vi "Calc_3-Ball-Conveyor_Module.vi"(0 "Enable":bool, 5 "Reset":bool, 7 "Grab Sensor":bool, 9 "Bottom Sensor":bool, 11 "Ball in Turret":bool=TRUE, 12 "Ball is out":bool) -> (4 "Motor Speed":dbl, 6 "Accepting Balls":bool, 8 "State":T1=enum."Holding 2", 10 "Ball Count":i32=2)   [LabVIEW 2012]
uses:
  3-Ball-Conveyor_Module_State.ctl
panel:
  in  "Slow":dbl=0.3
  in  "Fast":dbl=0.6
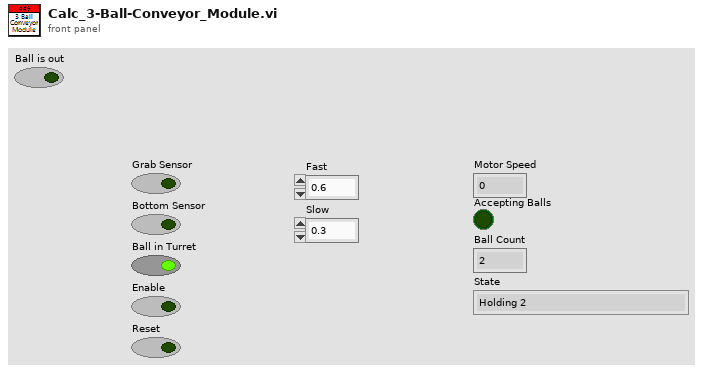
[diagram p1: front panel]
types:
  T1 = typedef "3-Ball-Conveyor_Module_State.ctl" = enum16{"No Balls", "Collecting Ball", "Holding 1", "Pushing Ball Out", "Holding 2", "Lowering Ball", "Reset", "Disabled"}
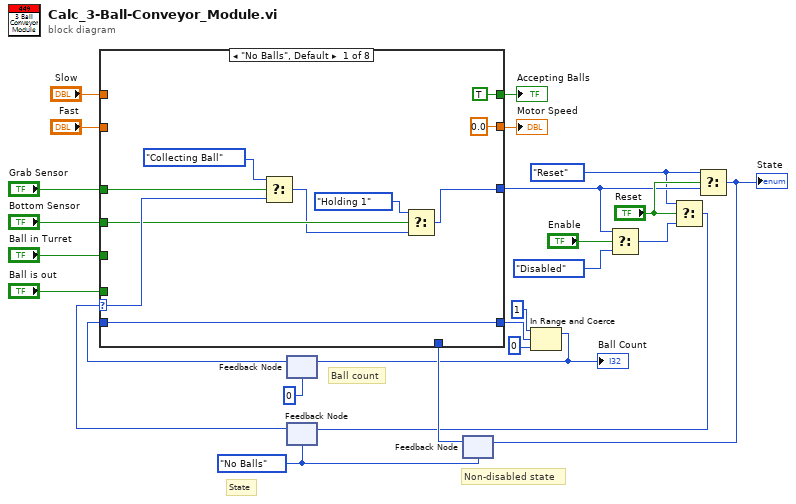
[diagram p0: block diagram]
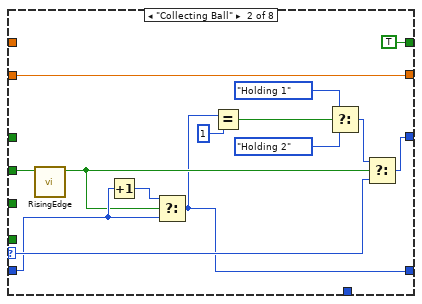
[diagram p2: hidden frame]
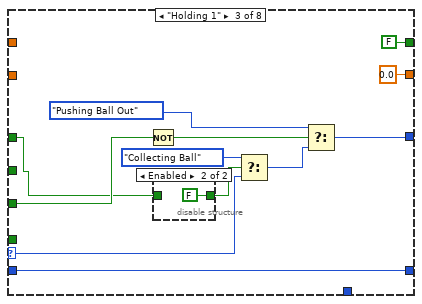
[diagram p3: hidden frame]
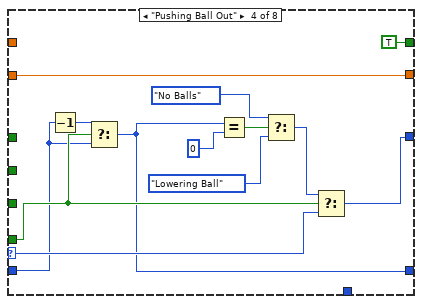
[diagram p5: hidden frame]
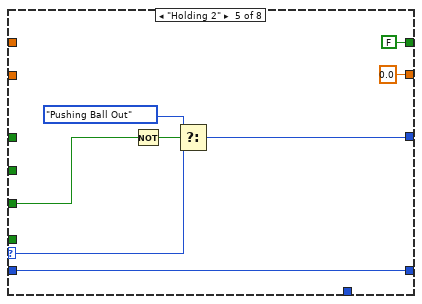
[diagram p6: hidden frame]
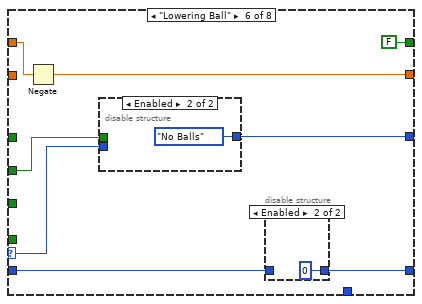
[diagram p7: hidden frame]
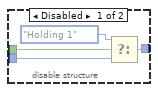
[diagram p8: hidden frame]
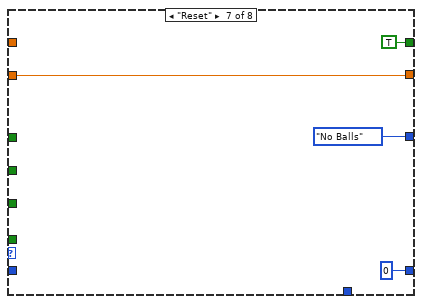
[diagram p10: hidden frame]
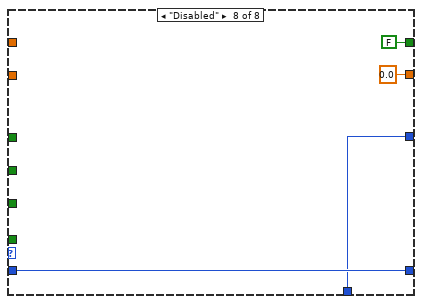
[diagram p11: hidden frame]
diagram:
  w6 = 3-Ball-Conveyor_Module_State."Reset"
  w11 = 3-Ball-Conveyor_Module_State."No Balls"
  # "Ball count"
  # "Non-disabled state"
  # "State"
  n1 = feedback #1(0) -> (w17:i32)
  n2 = feedback #2(w11) -> (w25:T1)
  n3 = feedback #3(w11) -> (w10:T1)
  n4 = case shown="\"No Balls\", Default" w25 {
    selector: w25 -> [w34 w46 w53 w74 w80 w88 _ _]
    tunnel: [0.0 ("Fast") w49 0.0 ("Fast") w76 0.0 ("Fast") w91 w103 0.0 ("Fast")] -> w24
    tunnel: [TRUE TRUE FALSE TRUE FALSE FALSE TRUE FALSE] -> w23
    tunnel: "Grab Sensor" -> [w35 _ w51 _ _ _ _ _]
    tunnel: [w26 w42 w59 w70 w81 w89 3-Ball-Conveyor_Module_State."No Balls" w104] -> w9
    tunnel: "Fast" -> [_ w49 _ w76 _ _ w103 _]
    tunnel: "Bottom Sensor" -> [w29 w47 _ _ _ w85 _ _]
    tunnel: "Ball in Turret" -> [_ _ w57 _ w82 _ _ _]
    tunnel: w17 -> [w31 w41 w56 w65 w79 w86 _ w105]
    tunnel: [w31 w36 w56 w64 w79 w87 0 ("t") w105] -> w4
    tunnel: "Slow" -> [_ _ _ _ _ w92 _ _]
    tunnel: w10 -> [_ _ _ _ _ _ _ w104]
    tunnel: "Ball is out" -> [_ _ _ w66 _ _ _ _]
    frame "No Balls", Default {
      n5 = Select(t=3-Ball-Conveyor_Module_State."Collecting Ball", s=w35, f=w34) -> (s? t:f=w28:T1)
      n6 = Select(t=3-Ball-Conveyor_Module_State."Holding 1", s=w29, f=w28) -> (s? t:f=w26:T1)
    }
    frame "Collecting Ball" {
      n7 = call "RisingEdge.vi"("BooleanIn"=w47) -> ("BooleanOut"=w40:bool)  [unwired: 10 in]
      n8 = Increment(x=w41) -> (x+1=w39:i32)
      n9 = Select(t=w39, s=w40, f=w41) -> (s? t:f=w36:i32)
      n10 = Equal?(x=w36, y=1) -> (x = y?=w44:bool)
      n11 = Select(t=3-Ball-Conveyor_Module_State."Holding 1", s=w44, f=3-Ball-Conveyor_Module_State."Holding 2") -> (s? t:f=w43:T1)
      n12 = Select(t=w43, s=w40, f=w46) -> (s? t:f=w42:T1)
    }
    frame "Holding 1" {
      n13 = Not(x=w57) -> (.not. x?=w58:bool)
      n14 = disable-structure shown="Enabled" {
        disable-tunnel: w51 -> [w62 _]
        disable-tunnel: [w62 FALSE ("Grab Sensor")] -> w50
        frame Disabled {
        }
        frame Enabled {
        }
      }
      n15 = Select(t=3-Ball-Conveyor_Module_State."Collecting Ball", s=w50, f=w53) -> (s? t:f=w54:T1)
      n16 = Select(t=3-Ball-Conveyor_Module_State."Pushing Ball Out", s=w58, f=w54) -> (s? t:f=w59:T1)
    }
    frame "Pushing Ball Out" {
      n17 = Decrement(x=w65) -> (x-1=w67:i32)
      n18 = Select(t=w67, s=w66, f=w65) -> (s? t:f=w64:i32)
      n19 = Equal?(x=w64, y=0) -> (x = y?=w72:bool)
      n20 = Select(t=3-Ball-Conveyor_Module_State."No Balls", s=w72, f=3-Ball-Conveyor_Module_State."Lowering Ball") -> (s? t:f=w71:T1)
      n21 = Select(t=w71, s=w66, f=w74) -> (s? t:f=w70:T1)
    }
    frame "Holding 2" {
      n22 = Not(x=w82) -> (.not. x?=w78:bool)
      n23 = Select(t=3-Ball-Conveyor_Module_State."Pushing Ball Out", s=w78, f=w80) -> (s? t:f=w81:T1)
    }
    frame "Lowering Ball" {
      n24 = Negate(x=w92) -> (-x=w91:dbl)
      n25 = disable-structure shown="Enabled" {
        disable-tunnel: [w96 3-Ball-Conveyor_Module_State."No Balls"] -> w89
        disable-tunnel: w88 -> [w95 _]
        disable-tunnel: w85 -> [w93 _]
        frame Disabled {
          n26 = Select(t=3-Ball-Conveyor_Module_State."Holding 1", s=w93, f=w95) -> (s? t:f=w96:T1)
        }
        frame Enabled {
        }
      }
      n27 = disable-structure shown="Enabled" {
        disable-tunnel: [w98 0] -> w87
        disable-tunnel: w86 -> [w98 _]
        frame Disabled {
        }
        frame Enabled {
        }
      }
    }
    frame "Reset" {
    }
    frame "Disabled" {
    }
  }
  "Motor Speed" <- w24
  "Accepting Balls" <- w23
  n28 = In Range and Coerce(upper limit=1, x=w4, lower limit=0 ("upper limit")) -> (coerced(x)=w1:i32)  [unwired: 1 out]
  "Ball Count" <- w1
  n29 = feedback-in #1(w1) -> ()
  n30 = Select(t=w9, s="Enable", f=3-Ball-Conveyor_Module_State."Disabled") -> (s? t:f=w14:T1)
  n31 = Select(t=w6, s="Reset", f=w14) -> (s? t:f=w8:T1)
  n32 = feedback-in #2(w8) -> ()
  n33 = Select(t=w6, s="Reset", f=w9) -> (s? t:f=w12:T1)
  "State" <- w12
  n34 = feedback-in #3(w12) -> ()
